vi "TCP-IP Mgr.Read-Write.vi"(6 "Rcv Q.Element":T1={"Cmd"="Task", "Sub"="TCP-IP Rcv", "Data1"=variant, "Data2"=variant}, 8 "error in":errorcluster, 9 "Q.Out":refnum<queue>, 10 "Q In":refnum<queue>, 11 "TCPIP ID":refnum<k5>) -> (0 "error out":errorcluster)   [LabVIEW 2017, in "TCP-IP Mgr.lvlib"]
uses:
  TCP-IP Mgr.lvlib
  <vilib>/KATE/Queues/Q.Element.ctl
  <vilib>/KATE/Queues/Queue Utils.lvlib
panel:
  out "Read Closed":bool
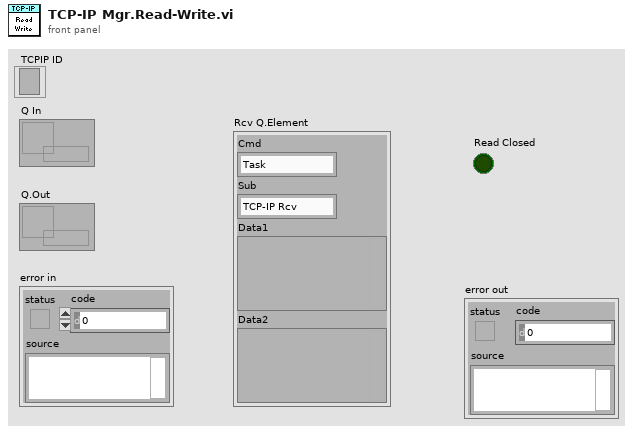
[diagram p1: front panel]
types:
  T1 = typedef "KATE_Lib.lvlib/Queue Utils.lvlib/Q.Element.ctl" = cluster{"Cmd":string, "Sub":string, "Data1":variant, "Data2":variant}
  T2 = enum16{"Standard", "Buffered", "CRLF", "Immediate"}
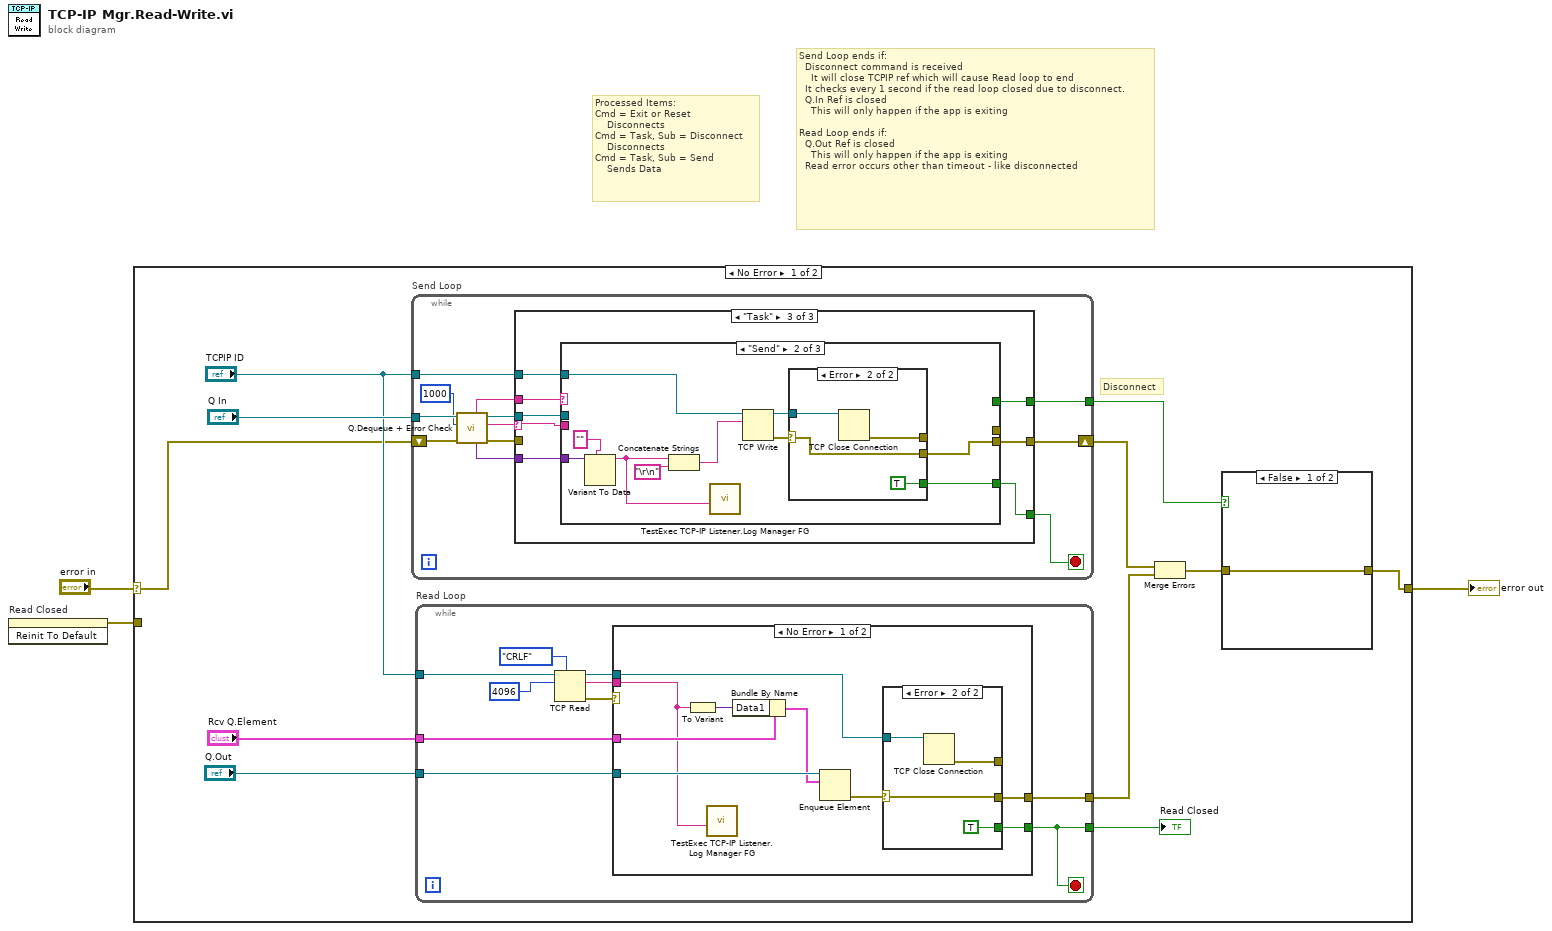
[diagram p0: block diagram]
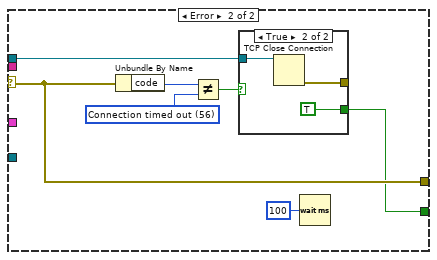
[diagram p4: hidden frame]
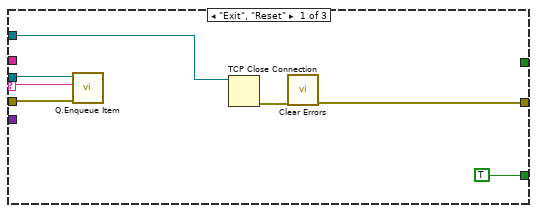
[diagram p6: hidden frame]
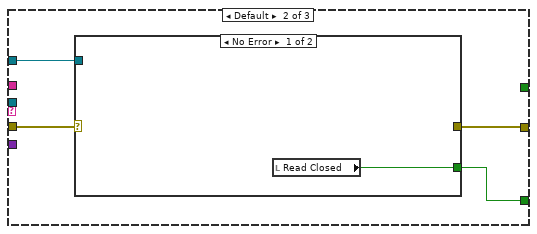
[diagram p7: hidden frame]
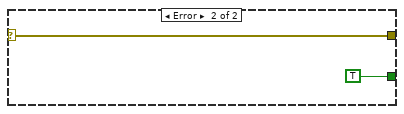
[diagram p8: hidden frame]
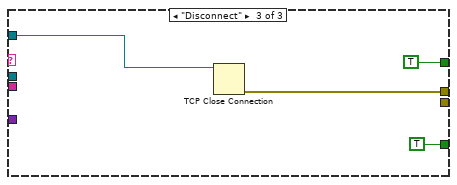
[diagram p11: hidden frame]
diagram:
  # "Send Loop ends if:\n  Disconnect command is received\n    It will close TCPIP ref which will cause Read loop to end\n  It checks every 1 second if the read loop closed due to disconnect.\n  Q.In Ref is closed\n    This will only happen if the app is exiting\n\nRead Loop ends if:\n  Q.Out Ref is closed\n    This will only happen if the app is exiting\n  Read error occurs other than timeout - like disconnected"
  # "Processed Items:\nCmd = Exit or Reset\n    Disconnects\nCmd = Task, Sub = Disconnect\n    Disconnects\nCmd = Task, Sub = Send\n    Sends Data"
  n1 = invoke on="Read Closed" class="Bool (strict)" method="Reinit To Default"() -> (error out=w1:errorcluster)  [unwired: 3 in, 2 out]
  n2 = case shown="No Error" "error in" {
    selector: "error in" -> [w11 w101]
    tunnel: [w5 w101] -> w3
    tunnel: w1 -> [_ _]
    frame No Error {
      # "Disconnect"
      n3 = while "Send Loop" {
        tunnel: "Q In" -> [w60]
        tunnel: "TCPIP ID" -> [w58]
        shift-right: [w54] -> w8
        shift-left: w11 -> [w55]
        tunnel: [w50] -> w9
        stop <- w53 stop-if-true
        n4 = call <vilib>:"Q.Dequeue + Error Check.vi"("Error In"=w55, "Timeout(-1)"=1000, "Q In"=w60) -> ("error out"=w56:errorcluster, "Cmd"=w59:string, "Q Out"=w57:refnum<queue>, "Data1"=w51:variant, "Sub"=w52:string)  [unwired: 3 in, 1 out]
        n5 = case shown="\"Task\"" w59 {
          selector: w59 -> [w65 _ w78]
          tunnel: w58 -> [w67 w69 w80]
          tunnel: w57 -> [w66 _ w79]
          tunnel: w56 -> [w64 w71 _]
          tunnel: [w62 w68 w77] -> w54
          tunnel: [TRUE w70 w76] -> w53
          tunnel: w52 -> [_ _ w82]
          tunnel: w51 -> [_ _ w81]
          tunnel: [_ _ w75] -> w50
          frame "Exit", "Reset" {
            n6 = call <vilib>:"Q.Enqueue Item.vi"("Error In"=w64, "Cmd"=w65, "Q In"=w66) -> ()  [unwired: 7 in, 2 out]
            n7 = TCP Close Connection(connection ID=w67) -> (error out=w63:errorcluster)  [unwired: 2 in, 1 out]
            n8 = call <vilib>:"Clear Errors.vi"("error in (no error)"=w63) -> ("error out"=w62:errorcluster)  [unwired: 5 in, 1 out]
          }
          frame Default {
            n9 = case shown="No Error" w71 {
              selector: w71 -> [_ w73]
              tunnel: [w72 TRUE] -> w70
              tunnel: w69 -> [_ _]
              tunnel: [_ w73] -> w68
              frame No Error {
                n10 = local read "Read Closed"() -> (w72:bool)
              }
              frame Error {
              }
            }
          }
          frame "Task" {
            n11 = case shown="\"Send\"" w82 {
              tunnel: w81 -> [_ w91 _]
              tunnel: w80 -> [_ w88 w100]
              tunnel: w79 -> [_ _ _]
              tunnel: w78 -> [_ _ _]
              tunnel: [_ w85 _] -> w77
              tunnel: [_ w84 TRUE] -> w76
              tunnel: [_ _ TRUE] -> w75
              tunnel: [_ _ w97] -> _
              frame Default {
                # "Ignore other tasks.\nShould not receive any"
              }
              frame "Send" {
                n12 = Variant To Data(type="", Variant=w91) -> (data=w83:string)  [unwired: 1 in, 1 out]
                n13 = Concatenate Strings(w83, "\r\n") -> (w89:string)
                n14 = call "TestExec TCP-IP Listener.Log Manager FG.vi"("Data"=w83) -> ()  [unwired: 11 in]
                n15 = TCP Write(connection ID=w88, data in=w89) -> (connection ID out=w86:refnum<k5>, error out=w87:errorcluster)  [unwired: 2 in, 1 out]
                n16 = case shown="Error" w87 {
                  selector: w87 -> [_ w95]
                  tunnel: w86 -> [_ w96]
                  tunnel: [_ w95] -> w85
                  tunnel: [_ TRUE] -> w84
                  tunnel: [_ w93] -> _
                  frame No Error {
                  }
                  frame Error {
                    n17 = TCP Close Connection(connection ID=w96) -> (error out=w93:errorcluster)  [unwired: 2 in, 1 out]
                  }
                }
              }
              frame "Disconnect" {
                n18 = TCP Close Connection(connection ID=w100) -> (error out=w97:errorcluster)  [unwired: 2 in, 1 out]
              }
            }
          }
        }
      }
      n19 = while "Read Loop" {
        tunnel: "TCPIP ID" -> [w24]
        tunnel: "Q.Out" -> [w21]
        tunnel: "Rcv Q.Element" -> [w19]
        tunnel: [w17] -> w7
        tunnel: [w16] -> w4
        stop <- w16 stop-if-true
        n20 = TCP Read(connection ID=w24, bytes to read=4096, 7:T2."CRLF" ("mode (standard)")) -> (connection ID out=w18:refnum<k5>, data out=w22:string, error out=w20:errorcluster)  [unwired: 2 in]
        n21 = case shown="No Error" w20 {
          selector: w20 -> [_ w40]
          tunnel: w22 -> [w26 _]
          tunnel: w21 -> [w34 _]
          tunnel: w19 -> [w32 _]
          tunnel: [w28 w40] -> w17
          tunnel: w18 -> [w29 w43]
          tunnel: [w27 w39] -> w16
          frame No Error {
            n22 = To Variant(anything=w26) -> (Variant=w31:variant)
            n23 = call "TestExec TCP-IP Listener.Log Manager FG.vi"("Data"=w26) -> ()  [unwired: 11 in]
            n24 = Bundle By Name(cluster=w32, "Data1"=w31) -> (w33:T1)
            n25 = Enqueue Element(queue=w34, element=w33) -> (error out=w30:errorcluster)  [unwired: 2 in, 2 out]
            n26 = case shown="Error" w30 {
              selector: w30 -> [_ w36]
              tunnel: w29 -> [_ w38]
              tunnel: [_ w36] -> w28
              tunnel: [_ TRUE] -> w27
              tunnel: [_ w35] -> _
              frame No Error {
              }
              frame Error {
                n27 = TCP Close Connection(connection ID=w38) -> (error out=w35:errorcluster)  [unwired: 2 in, 1 out]
              }
            }
          }
          frame Error {
            w45 = 56 items=["No Error", "Argument Error", "Memory Full", "Out of Zone", "End of File", "File Already Open", "Generic File IO Error", "File Not Found", "File Permission Error", "Disk Full", "Duplicate Path", "Too Many Files Open", "Not Enabled", "Resource File Not Found", "Cannot Add Resource", "Resource Not Found", "Image Not Found", "Image Memory Error", "Pen Does Not Exist", "Config Bad Type", "Config Token Not Found", "Config Parse Error", "Config Memory Error", "Bad External Code Format", "Bad External Code Offset", "External Code Not Present", "Null Window", "Destroy Window Mixup", "Null Menu", "Print Aborted", "Bad Print Record", "Print Driver Error", "Windows Error During Print", "Memory Error During Print", "Print Dialog Error", "Generic Print Error", "Invalid Device Refnum", "Device Not Found", "Device Parameter Error", "Device Unit Error", "Can't Open Device", "Device Call Aborted", "Generic Error", "Cancelled By User", "Object ID Too Low", "Object ID Too High", "Object Not In Heap", "Unknown Heap", "Bad DefProc ID", "DefProc Not In Table", "Message Out Of Range", "Null Method", "Unknown Message", "Manager Call Not Supported", "Bad address", "Connection In progress", "Connection timed out", "Connection is already in progress", "Network attribute not supported", "Network error", "Address in use", "System out of memory", "Connection aborted", "Connection refused", "Connection is not connected", "Connection is already connected", "Connection closed", "Initialize error (interapplication manager)", "Bad occurrence", "Wait on unbound occurrence handler", "Occurrence queue overflow", "Bad path", "Semaphore not signaled", "Unrecognized type (interapplication manager)"] ("2nd Error to Convert")
            n28 = Unbundle By Name(w40) -> ("code"=w44:i32)
            n29 = Not Equal?(x=w44, y=w45) -> (x != y?=w42:bool)
            n30 = case shown="True" w42 {
              tunnel: w43 -> [_ w48]
              tunnel: [_ TRUE] -> w39
              tunnel: [_ w46] -> _
              frame False {
              }
              frame True {
                n31 = TCP Close Connection(connection ID=w48) -> (error out=w46:errorcluster)  [unwired: 2 in, 1 out]
              }
            }
            n32 = Wait (ms)(milliseconds to wait=u32 100) -> ()  [unwired: 1 out]
          }
        }
      }
      "Read Closed" <- w4
      n33 = Merge Errors(w8, w7) -> (w6:errorcluster)
      n34 = case shown="False" w9 {
        tunnel: w6 -> [w15 _]
        tunnel: [w15 _] -> w5
        frame False {
        }
        frame True {
        }
      }
    }
    frame Error {
    }
  }
  "error out" <- w3
